vi "Copy SM Template.vi"(11 "Refs In":T1) -> (0 "error out":errorcluster, 3 "Refs":T1)   [LabVIEW 2022 SP3, in "FlexBlocks Support.lvlib"]
uses:
  FlexBlocks Support.lvlib
  SM Refs.ctl
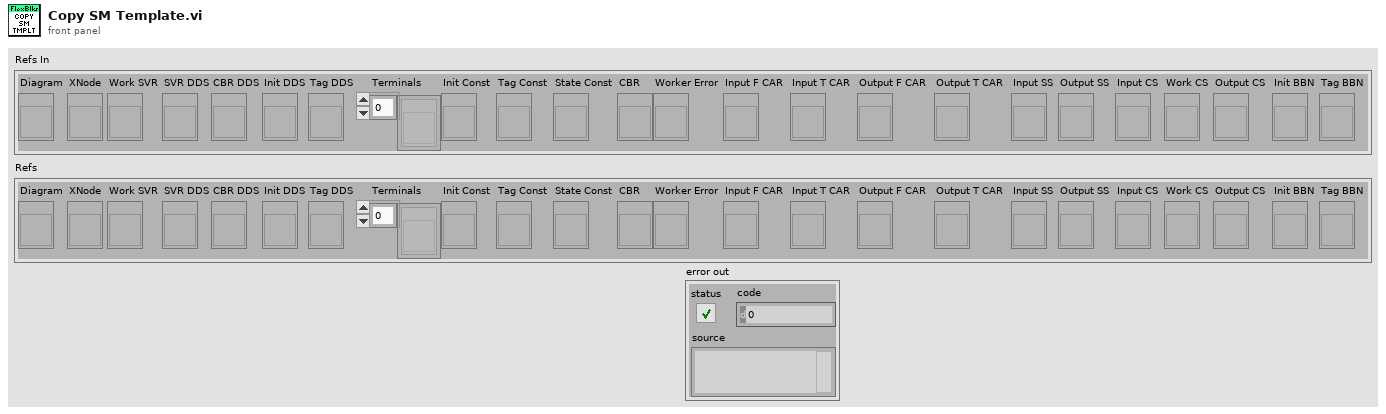
[diagram p1: front panel]
types:
  T1 = typedef "FlexBlocks Support.lvlib/SM Refs.ctl" = cluster{"Diagram":refnum<vi>, "XNode":refnum<vi>, "Work SVR":refnum<vi>, "SVR DDS":refnum<vi>, "CBR DDS":refnum<vi>, "Init DDS":refnum<vi>, "Tag DDS":refnum<vi>, "Terminals":refnum<vi>[], "Init Const":refnum<vi>, "Tag Const":refnum<vi>, "State Const":refnum<vi>, "CBR":refnum<vi>, "Worker Error":refnum<vi>, "Input F CAR":refnum<vi>, "Input T CAR":refnum<vi>, "Output F CAR":refnum<vi>, "Output T CAR":refnum<vi>, "Input SS":refnum<vi>, "Output SS":refnum<vi>, "Input CS":refnum<vi>, "Work CS":refnum<vi>, "Output CS":refnum<vi>, "Init BBN":refnum<vi>, "Tag BBN":refnum<vi>}
  T2 = typedef "FlexBlocks Support.lvlib/Paths.ctl" = cluster{"FlexBlocks":path, "Workers Root":path, "Specialized Editors":path, "Worker Template":path, "SM Template":path, "Read Control Value Vim":path, "Write Indicator Value Vim":path}
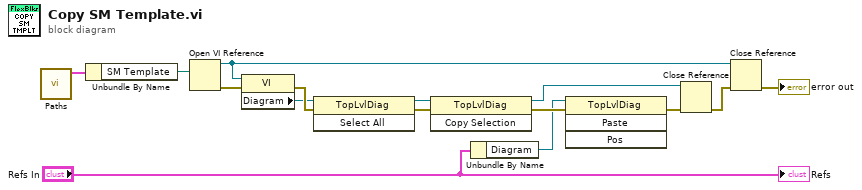
[diagram p0: block diagram]
diagram:
  n1 = call "Paths.vi"() -> ("Paths"=w14:T2)  [unwired: 11 in]
  n2 = Unbundle By Name(w14) -> ("SM Template"=w13:path)
  n3 = Open VI Reference(vi path=w13) -> (vi reference=w3:refnum<vi>, error out=w12:errorcluster)  [unwired: 5 in]
  n4 = property class="VI"(reference=w3, error in=w12) -> (error out=w15:errorcluster, "Diagram"=w11:refnum<vi>)  [unwired: 1 out]
  n5 = invoke class="TopLvlDiag" method="Select All"(reference=w11, error in=w15) -> (reference out=w10:refnum<vi>, error out=w9:errorcluster)  [unwired: 1 in, 1 out]
  n6 = invoke class="TopLvlDiag" method="Copy Selection"(reference=w10, error in=w9) -> (reference out=w5:refnum<vi>, error out=w7:errorcluster)  [unwired: 1 in, 1 out]
  n7 = Unbundle By Name("Refs In") -> ("Diagram"=w4:refnum<vi>)
  n8 = invoke class="TopLvlDiag" method="Paste"(reference=w4, error in=w7) -> (error out=w6:errorcluster)  [unwired: 2 in, 3 out]
  n9 = Close Reference(reference=w5, error in (no error)=w6) -> (error out=w2:errorcluster)
  n10 = Close Reference(reference=w3, error in (no error)=w2) -> (error out=→"error out":errorcluster)
  "Refs" <- "Refs In"
